vi "Parse Project TargetItem Name.vi"(11 "project targetitem name":string) -> (0 "find fpga & create target struct, unless exists already":bool, 1 "create fpga, unless exists already":bool, 2 "no menu":bool, 3 "use owner menu":bool)   [LabVIEW 2020, in "NI_TargetHelper.lvlib"]
uses:
  <vilib>/TargetSupport/NI_TargetHelper/NI_TargetHelper.lvlib
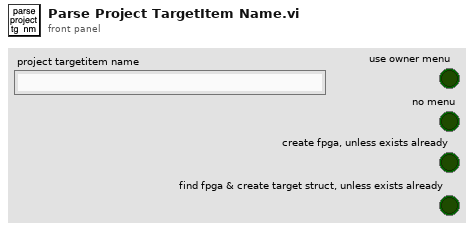
[diagram p1: front panel]
types:
  T1 = cluster{"name":string, "owner":bool, "none":bool, "one":bool, "auto":bool, "choose":bool, "opt#":bool, "ipaddr":bool, "[loc,]mod":bool, "TSname":string}[]
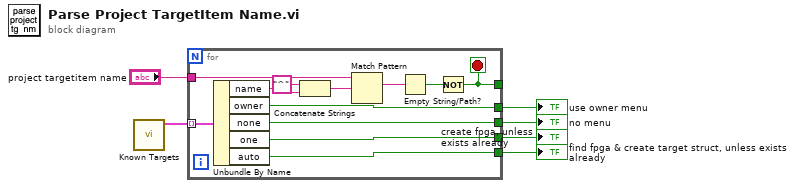
[diagram p0: block diagram]
diagram:
  n1 = call <vilib>:"Known Targets.vi"() -> ("targets        project targetItem name              menu to use                    fpga sub                                           suffix info"=w6:T1)  [unwired: 11 in]
  n2 = for {
    tunnel: w6 -> [w18] mode=indexing
    tunnel: "project targetitem name" -> [w15]
    tunnel: [w11] -> _
    tunnel: [w10] -> w4
    tunnel: [w9] -> w3
    tunnel: [w8] -> w2
    tunnel: [w7] -> w1
    stop <- w11 stop-if-true
    n3 = Unbundle By Name(w18) -> ("name"=w14:string, "owner"=w10:bool, "none"=w9:bool, "one"=w8:bool, "auto"=w7:bool)
    n4 = Concatenate Strings("^" ("string"), w14) -> (w16:string)
    n5 = Match Pattern(string=w15, regular expression=w16) -> (match substring=w13:string)  [unwired: 1 in, 3 out]
    n6 = Empty String/Path?(string/path=w13) -> (empty?=w12:bool)
    n7 = Not(x=w12) -> (.not. x?=w11:bool)
  }
  "use owner menu" <- w4
  "no menu" <- w3
  "create fpga, unless exists already" <- w2
  "find fpga & create target struct, unless exists already" <- w1
